vi "AutoTouchDataWire.vi"(11 "String":string) -> (3 "result":string="N/A")   [LabVIEW 2015]
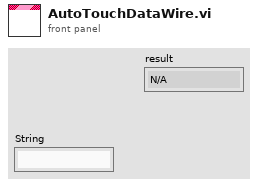
[diagram p1: front panel]
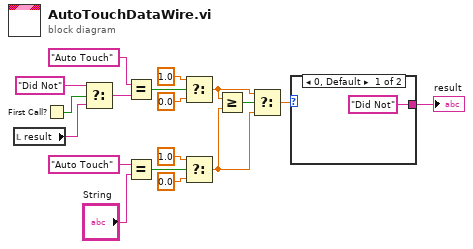
[diagram p0: block diagram]
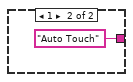
[diagram p2: hidden frame]
diagram:
  n1 = local read "result"() -> (w4:string)
  n2 = First Call?() -> (First Call?: T/F=w6:bool)
  n3 = Select(t="Did Not" ("x"), s=w6, f=w4) -> (s? t:f=w3:string)
  n4 = Equal?(x="Auto Touch", y=w3) -> (x = y?=w14:bool)
  n5 = Equal?(x="Auto Touch", y="String") -> (x = y?=w8:bool)
  n6 = Select(t=1.0, s=w14, f=0.0) -> (s? t:f=w2:dbl)
  n7 = Select(t=1.0, s=w8, f=0.0) -> (s? t:f=w1:dbl)
  n8 = Greater Or Equal?(x=w2, y=w1) -> (x >= y?=w16:bool)
  n9 = Select(t=w2, s=w16, f=w1) -> (s? t:f=w17:dbl)
  n10 = case shown="0, Default" w17 {
    tunnel: ["Did Not" ("x") "Auto Touch" ("x")] -> w18
    frame 0, Default {
    }
    frame 1 {
    }
  }
  "result" <- w18
